vi "Generate SR No.vi"(8 "error in (no error)":errorcluster, 11 "Table Control":string[][](table)) -> (0 "error out":errorcluster, 3 "output Table":string[][](array[string]))   [LabVIEW 2018]
panel:
  out "SR NO Numeric":i32[](array[numeric])
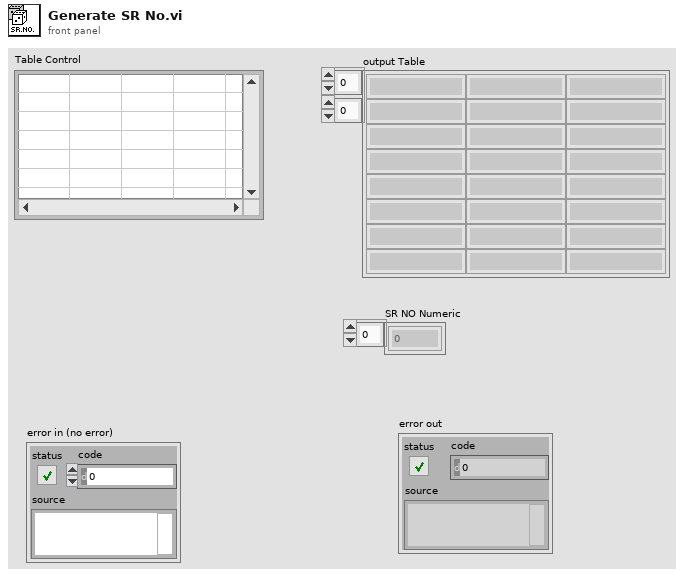
[diagram p1: front panel]
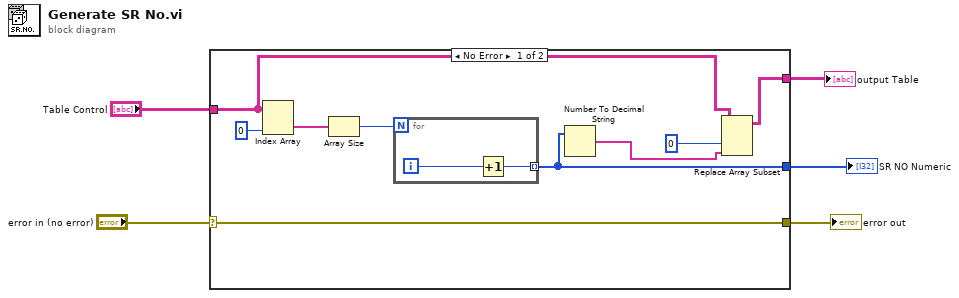
[diagram p0: block diagram]
diagram:
  n1 = case shown="No Error" "error in (no error)" {
    selector: "error in (no error)" -> [w12 w17]
    tunnel: "Table Control" -> [w8 w18]
    tunnel: [w9 w18] -> w4
    tunnel: [w12 w17] -> w2
    tunnel: [w11 _] -> w1
    frame No Error {
      n2 = Index Array(array=w8, index (col)=0 ("Coloumn No")) -> (element=w14:string[])  [unwired: 1 in]
      n3 = Array Size(array=w14) -> (size(s)=w13:i32)
      n4 = for {
        N: w13 -> [_]
        tunnel: [w15] -> w11 mode=indexing
        i -> [w16]
        n5 = Increment(x=w16) -> (x+1=w15:i32)
      }
      n6 = Number To Decimal String(number=w11) -> (decimal integer string=w6:string[])  [unwired: 1 in]
      n7 = Replace Array Subset(array=w8, new element=w6, index (col)=0 ("disabled index (col)")) -> (w9:string[][])  [unwired: 1 in]
    }
    frame Error {
    }
  }
  "output Table" <- w4
  "error out" <- w2
  "SR NO Numeric" <- w1
